vi "Get Description.vi"(8 "error in (no error)":errorcluster, 11 "CIPC Reference":u64) -> (0 "error out":errorcluster, 3 "Description":string)   [LabVIEW 2021, in "CIF_NI_CIPC.lvlib"]
uses:
  CIF_NI_CIPC.lvlib
  SubVIs/Check Error Core.vi
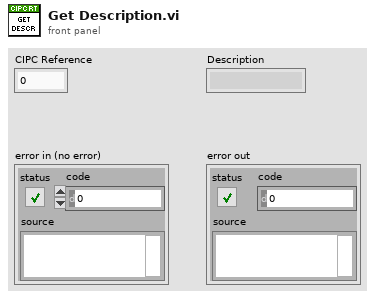
[diagram p1: front panel]
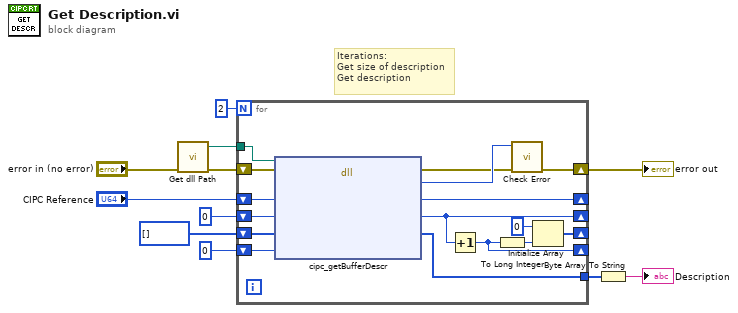
[diagram p0: block diagram]
diagram:
  # "Iterations:\nGet size of description\nGet description"
  n1 = call "Get dll Path.vi"() -> ("appended path"=w4:path)  [unwired: 5 in]
  n2 = for {
    N: 2 -> [_]
    tunnel: w4 -> [w12]
    shift-right: [w23] -> _
    shift-left: "CIPC Reference" -> [w15]
    shift-right: [w24] -> w3
    shift-left: "error in (no error)" -> [w14]
    shift-right: [w17] -> _
    shift-left: u8[] [] ("initialized array") -> [w16]
    shift-right: [w19] -> _
    shift-left: u32 0 ("descr_size") -> [w21]
    shift-right: [w18] -> _
    shift-left: u32 0 ("el_descr_maxsize") -> [w22]
    tunnel: [w11] -> w2
    n3 = dll-call lib="libnicipc.*" fn="cipc_getBufferDescr"(path in=w12, error in=w14, "cipc_buffer_ref"=w15, "descr_size"=w21, "el_descr"=w16, "el_descr_maxsize"=w22) -> (error out=w25:errorcluster, "return type"=w26:i32, "cipc_buffer_ref"=w23:u64, "descr_size"=w19:u32, "el_descr"=w11:u8[])  [unwired: 2 in, 1 out]
    n4 = Increment(x=w19) -> (x+1=w18:u32)
    n5 = To Long Integer(number=w18) -> (32bit integer=w13:i32)
    n6 = call "Check Error.vi"("error in (no error)"=w25, "Error Code"=w26) -> ("error out"=w24:errorcluster)  [unwired: 9 in]
    n7 = Initialize Array(u8 0, w13) -> (w17:u8[])
  }
  "error out" <- w3
  n8 = Byte Array To String(unsigned byte array=w2) -> (string=→"Description":string)
